vi "Start.vi"(8 "Error In":errorcluster, 11 "object in":refnum<class "IInstrument Base.lvclass">) -> (0 "Error Out":errorcluster, 3 "object out":refnum<class "IInstrument Base.lvclass">)   [LabVIEW 2023, in "IInstrument Base.lvclass"]
uses:
  IInstrument Base.lvclass
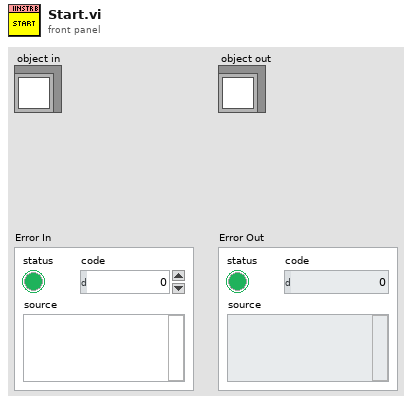
[diagram p1: front panel]
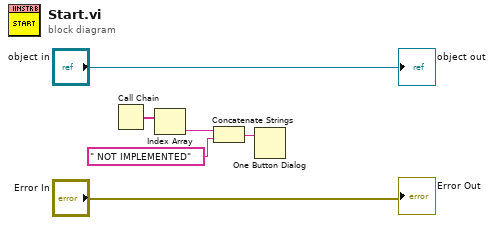
[diagram p0: block diagram]
diagram:
  n1 = Call Chain() -> (call chain=w4:string[])
  n2 = Index Array(array=w4) -> (element=w1:string)  [unwired: 1 in]
  n3 = Concatenate Strings(w1, " NOT IMPLEMENTED" ("string")) -> (w3:string)
  n4 = One Button Dialog(message=w3) -> ()  [unwired: 1 in, 1 out]
  "Error Out" <- "Error In"
  "object out" <- "object in"
